vi "HENES.vi"() -> ()   [LabVIEW 2024]
uses:
  <vilib>/Python/Open Venv Python Session.vi
  <vilib>/vision/NI_Vision_Development_Module.lvlib
  <vilib>/vision/driver/NI_Vision_Acquisition_Software.lvlib
  <vilib>/userDefined/High Color/IMAQdx.ctl
panel:
  in  "Session In":T1
  out "error out 2":errorcluster
  out "error out":errorcluster
  out "return value":string
  out "python_error":errorcluster
  out "Image":T2(plugin-control)
  out "R Pixels":u8[][](array[numeric])
  out "G Pixels":u8[][](array[numeric])
  out "B Pixels":u8[][](array[numeric])
  in  "ROI Descriptor":T3={"Global Rectangle"=[305, 202, 665, 606], "Contours"=[{"ID"=enum."External", "Type"=3, "Coordinates"=[305, 202, 665, 606]}]} {"Contours"."Type" items=["No Selection", "Point", "Line", "Rectangle", "Oval", "Polygon", "Freehand Region", "Annulus", "Unused2", "Unused3", "Broken Line", "Freehand Line", "Rotated Rectangle"]}
  in  "stop":bool
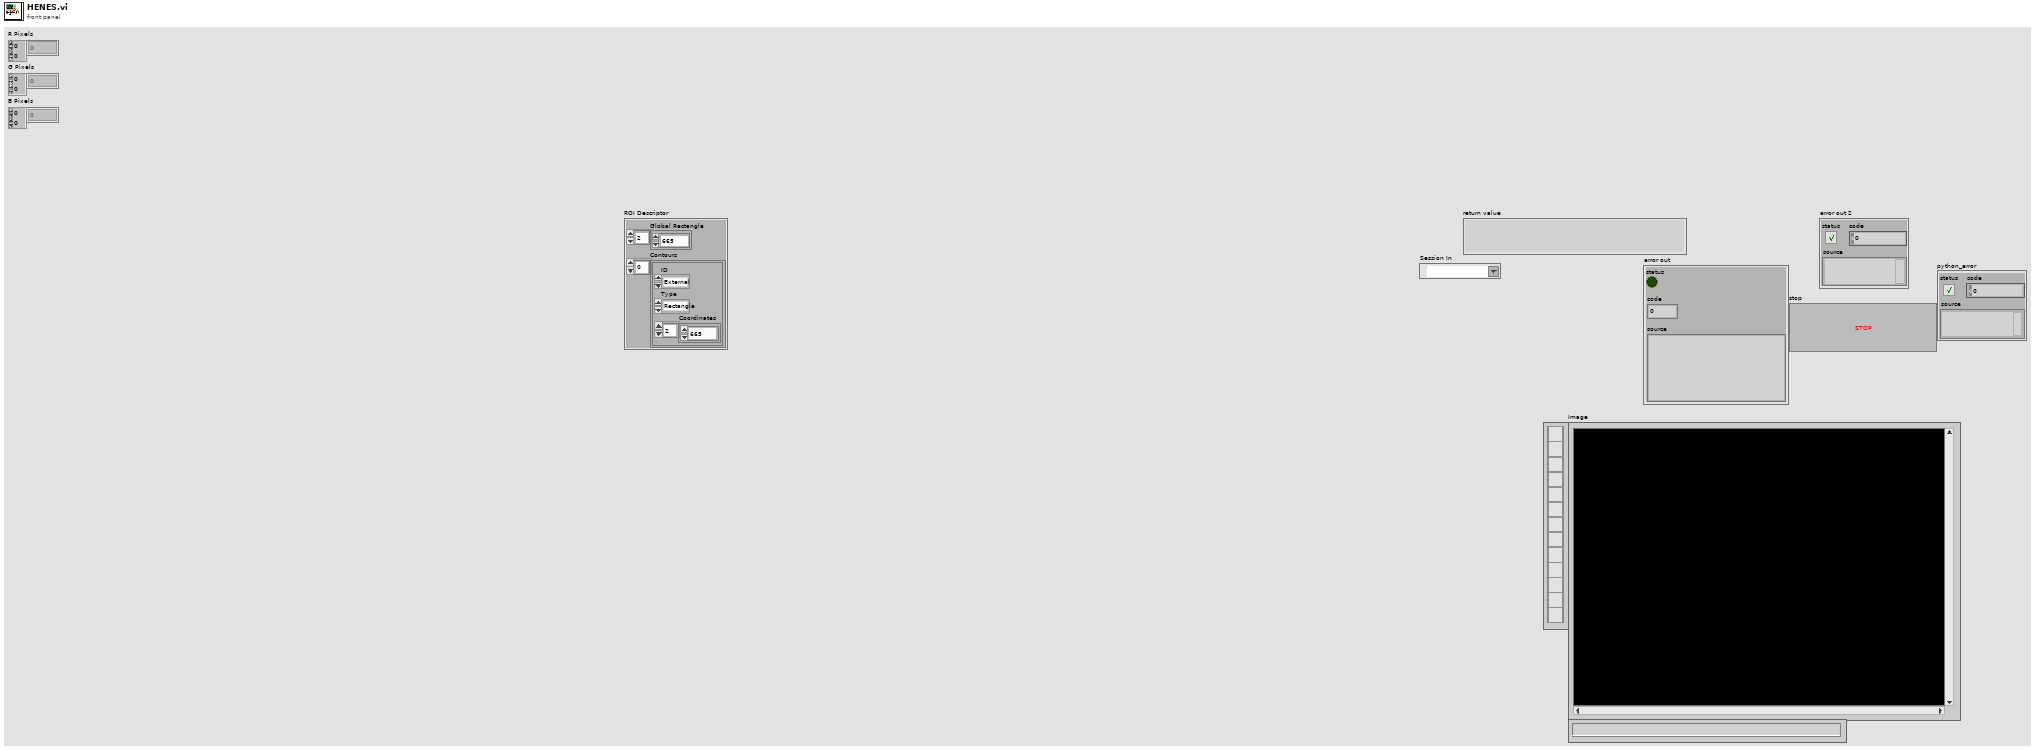
[diagram p1: front panel]
types:
  T1 = typedef "IMAQdx.ctl" = refnum<k21>
  T2 = typedef "IMAQ Image.ctl" = refnum<image>
  T3 = cluster{"Global Rectangle":i32[], "Contours":cluster{"ID":enum32{"External", "Internal"}, "Type":u32, "Coordinates":i32[]}[]}
  T4 = cluster{"Origin Pixel":cluster{"X":sgl, "Y":sgl}, "X Axis Pixel":cluster{"X":sgl, "Y":sgl}, "Axis Reference":u32}
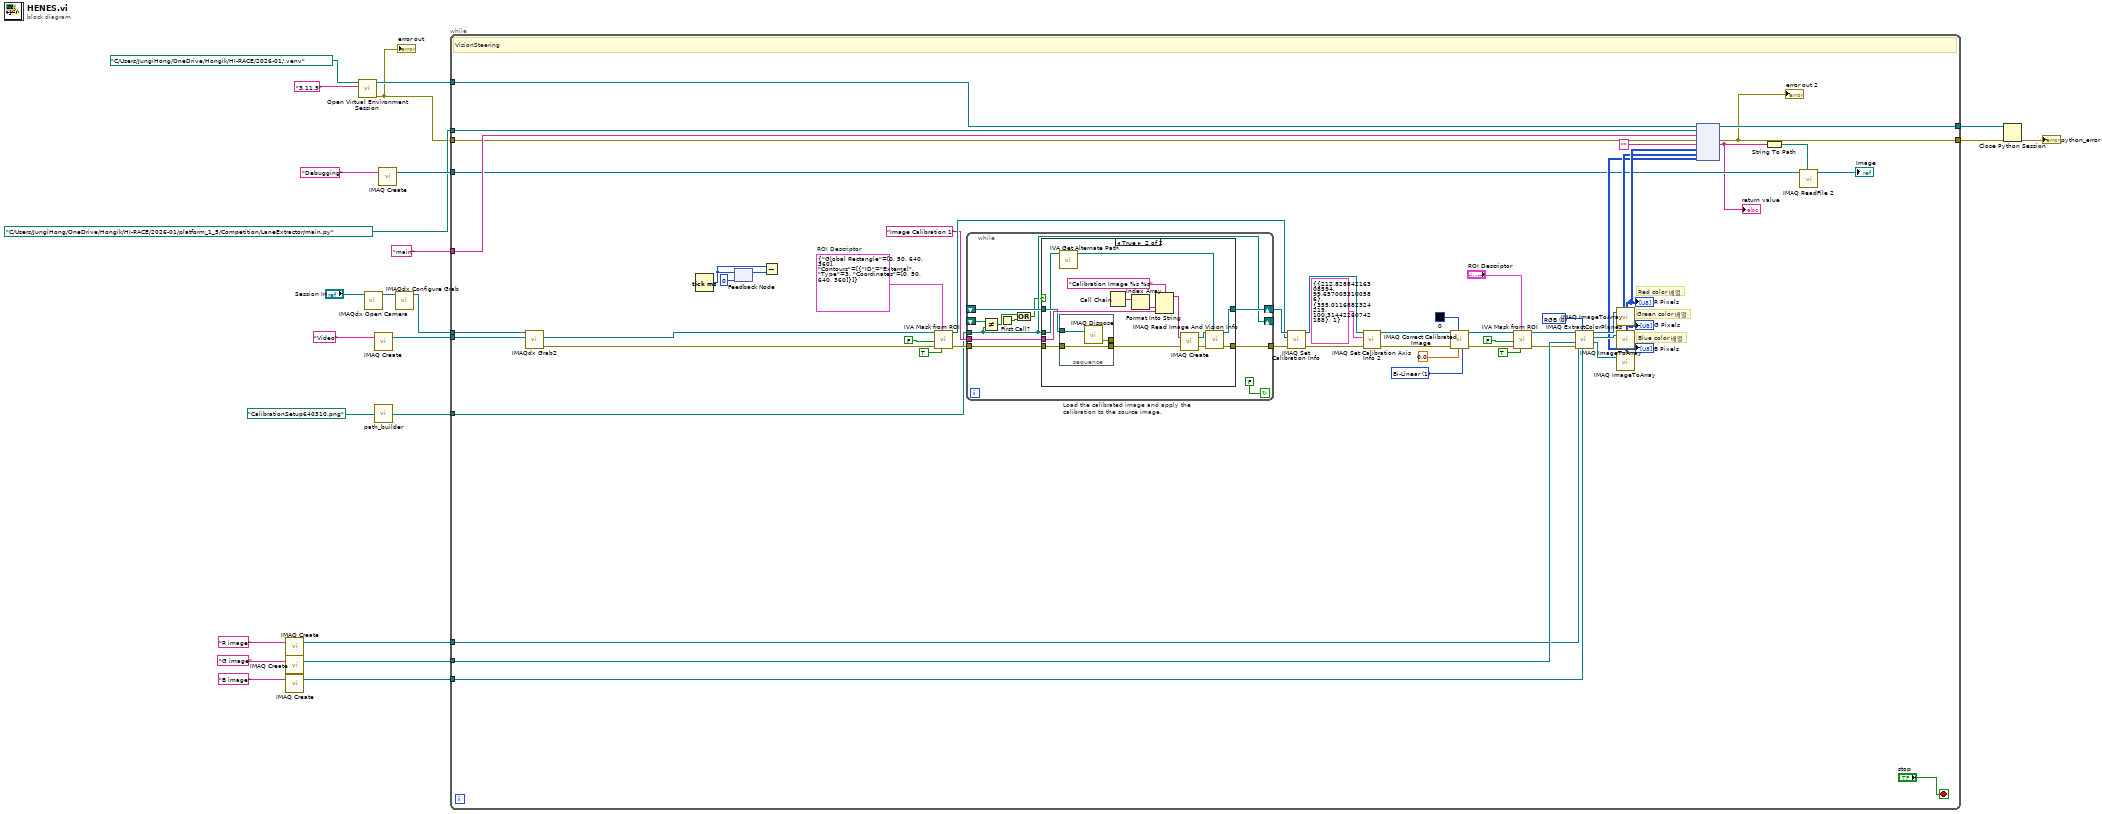
[diagram p0: block diagram]
diagram:
  n1 = call "IMAQ Create"("Image Name"="R image") -> ("New Image"=w9:T2)  [unwired: 4 in, 1 out]
  n2 = call "IMAQ Create"("Image Name"="G image") -> ("New Image"=w10:T2)  [unwired: 4 in, 1 out]
  n3 = call "IMAQ Create"("Image Name"="B image") -> ("New Image"=w11:T2)  [unwired: 4 in, 1 out]
  n4 = call-poly <vilib>:"Open Virtual Environment Session.vi"("Python version"="3.11.9", "Env path"=path "C:/Users/JungiHong/OneDrive/Hongik/HI-RACE/2026-01/.venv") -> ("error out"=w4:errorcluster, "session out"=w20:refnum<k35>)  [unwired: 8 in]
  "error out" <- w4
  n5 = call <vilib>:"IMAQdx Open Camera.vi"("Session In"="Session In") -> ("Session Out"=w2:T1)  [unwired: 9 in, 1 out]
  n6 = call "IMAQ Create"("Image Name"="Video") -> ("New Image"=w23:T2)  [unwired: 4 in, 1 out]
  n7 = call "path_builder.vi"("Name"=path "CalibrationSetup640310.png") -> ("appended path"=w22:path)
  n8 = call "IMAQ Create"("Image Name"="Debugging") -> ("New Image"=w15:T2)  [unwired: 4 in, 1 out]
  n9 = call <vilib>:"IMAQdx Configure Grab.vi"("Session In"=w2) -> ("Session Out"=w1:T1)  [unwired: 9 in, 1 out]
  n10 = while {
    tunnel: w23 -> [w27]
    tunnel: w22 -> [w54]
    tunnel: w20 -> [w51]
    tunnel: [w50] -> w17
    tunnel: w15 -> [w32]
    tunnel: w11 -> [w44]
    tunnel: w10 -> [w43]
    tunnel: w9 -> [w42]
    tunnel: path "C:/Users/JungiHong/OneDrive/Hongik/HI-RACE/2026-01/platform_1_5/Competition/LaneExtractor/main.py" ("module in") -> [w37]
    tunnel: "main" ("module out") -> [w36]
    tunnel: w4 -> [w35]
    tunnel: [w33] -> w6
    tunnel: w1 -> [w28]
    stop <- "stop" stop-if-true
    w45 = u16 0 items=["RGB", "HSL", "HSV", "HSI"] ("Color Mode")
    w62 = u32 1 items=["Zero Order", "Bi-Linear", "Quadratic", "Cubic Spline"] ("Interpolation Type")
    w74 = T3 {"Global Rectangle"=[0, 50, 640, 360], "Contours"=[{"ID"=enum."External", "Type"=3, "Coordinates"=[0, 50, 640, 360]}]}  # ROI Descriptor
    # "Blue color 배열"
    # "Green color 배열"
    # "Red color 배열"
    # "VisionSteering"
    n11 = call <vilib>:"IMAQdx Grab2.vi"("Image In"=w27, "Session In"=w28) -> ("error out"=w25:errorcluster, "Image Out"=w26:T2)  [unwired: 6 in, 2 out]
    n12 = Tick Count (ms)() -> (millisecond timer value=w77:u32)
    n13 = feedback #1(u32 0 ("millisecond timer value")) -> (w76:u32)
    n14 = feedback-in #1(w77) -> ()
    n15 = Subtract(x=w77, y=w76) -> ()  [unwired: 1 out]
    n16 = call <vilib>:"IVA Mask from ROI.vi"("Shrink"=TRUE, "ROI Descriptor"=w74, "error in (no error)"=w25, "Out / In"=FALSE, "Image Src"=w26) -> ("error out"=w71:errorcluster, "Image Out"=w67:T2)  [unwired: 5 out]
    n17 = while "Load the calibrated image and apply the calibration to the source image." {
      shift-right: [w88] -> w70
      shift-left: _ -> [w87]
      tunnel: [w85] -> w69
      tunnel: w71 -> [w84]
      tunnel: w54 -> [w81]
      tunnel: "Image Calibration 1" ("Step Name") -> [w83]
      shift-right: [w81] -> _
      shift-left: _ -> [w82]
      stop <- FALSE continue-if-true
      n18 = Not Equal?(x=w82, y=w81) -> (x != y?=w79:bool)
      n19 = First Call?() -> (First Call?: T/F=w80:bool)
      n20 = Or(x=w79, y=w80) -> (x .or. y?=w78:bool)
      n21 = case shown="True" w78 {
        tunnel: [w90 w102] -> w88
        tunnel: w87 -> [w90 w94]
        tunnel: [w89 w99] -> w85
        tunnel: w84 -> [w89 w95]
        tunnel: w81 -> [_ w92]
        tunnel: w83 -> [_ w96]
        frame False {
        }
        frame True {
          n22 = call <vilib>:"IVA Get Alternate Path.vi"("Path In"=w92) -> ("Path Out"=w91:path)  [unwired: 10 out]
          n23 = stacked-sequence {
            tunnel: w95 -> [w106]
            tunnel: w94 -> [w107]
            tunnel: [w106] -> w93
            tunnel: [w105] -> _
            frame #0 {
              n24 = call "IMAQ Dispose"("Image"=w107) -> ("error out"=w105:errorcluster)  [unwired: 2 in, 3 out]
            }
          }
          n25 = Call Chain() -> (call chain=w98:string[])
          n26 = Index Array(array=w98) -> (element=w97:string)  [unwired: 1 in]
          n27 = Format Into String(format string="Calibration Image %s %s" ("Image Name"), w97, w96) -> (resulting string=w104:string)  [unwired: 2 in, 1 out]
          n28 = call "IMAQ Create"("Image Name"=w104, "error in (no error)"=w93) -> ("New Image"=w101:T2, "error out"=w100:errorcluster)  [unwired: 2 in, 1 out]
          n29 = call "IMAQ Read Image And Vision Info"("File Path"=w91, "error in (no error)"=w100, "Image"=w101) -> ("error out"=w99:errorcluster, "Image Out"=w102:T2)  [unwired: 1 in, 6 out]
        }
      }
    }
    n30 = call "IMAQ Set Calibration Info"("error in (no error)"=w69, "Image Dst"=w67, "Image Src"=w70) -> ("error out"=w68:errorcluster, "Calibrated Image"=w64:T2)  [unwired: 1 in, 6 out]
    n31 = call-poly "IMAQ Set Calibration Axis Info 2"("error in (no error)"=w68, "Calibration Axis Info"=T4 {"Origin Pixel"={"X"=212.82884, "Y"=99.657005}, "X Axis Pixel"={"X"=355.0117, "Y"=100.31442}, "Axis Reference"=1}, "Calibration Template Image In"=w64) -> ("error out"=w65:errorcluster, "Calibration Template Image Out"=w60:T2)  [unwired: 7 out]
    n32 = call "IMAQ Correct Calibrated Image"("Interpolation Type"=w62, "Replace Value"=sgl 0.0, "Color Replace Value"=u32 0, "error in (no error)"=w65, "Image Src"=w60) -> ("error out"=w61:errorcluster, "Corrected Image"=w52:T2)  [unwired: 2 in, 3 out]
    n33 = call <vilib>:"IVA Mask from ROI.vi"("Shrink"=TRUE, "ROI Descriptor"="ROI Descriptor", "error in (no error)"=w61, "Out / In"=FALSE, "Image Src"=w52) -> ("error out"=w34:errorcluster, "Image Out"=w41:T2)  [unwired: 5 out]
    n34 = call "IMAQ ExtractColorPlanes"("Blue or Luma or Val or Inten Plane"=w44, "Color Mode"=w45, "error in (no error)"=w34, "Green or Sat Plane"=w43, "Red or Hue Plane"=w42, "Image Src"=w41) -> ("Blue or Luma or Val or Inten Plane out"=w48:T2, "Green or Sat Plane out"=w47:T2, "Red or Hue Plane out"=w46:T2)  [unwired: 2 in, 1 out]
    n35 = call "IMAQ ImageToArray"("Image"=w46) -> ("Image Pixels (U8)"=w40:u8[][])  [unwired: 3 in, 4 out]
    "R Pixels" <- w40
    n36 = call "IMAQ ImageToArray"("Image"=w47) -> ("Image Pixels (U8)"=w39:u8[][])  [unwired: 3 in, 4 out]
    "G Pixels" <- w39
    n37 = call "IMAQ ImageToArray"("Image"=w48) -> ("Image Pixels (U8)"=w38:u8[][])  [unwired: 3 in, 4 out]
    "B Pixels" <- w38
    n38 = node(w51, w37, w36, w35, "", w40, w39, w38) -> (w50:refnum<k35>, w33:errorcluster, w30:string)  [unwired: 3 in, 2 out]
    "return value" <- w30
    "error out 2" <- w33
    n39 = String To Path(string=w30) -> (path=w29:path)
    n40 = call "IMAQ ReadFile 2"("File Path"=w29, "Image"=w32) -> ("Image Out"=→"Image":T2)  [unwired: 5 in, 4 out]
  }
  n41 = Close Python Session(session in=w17, error in=w6) -> (11:→"python_error":errorcluster)
